vi "Get Server Certificate (Server).vi"(10 "Server Certificates":T1) -> (2 "server certificate file":path)   [LabVIEW 2013, in "OPC UA runtime.lvclass"]
doc: "Get server certificate for OPC UA server connection."
uses:
  OPC UA runtime.lvclass
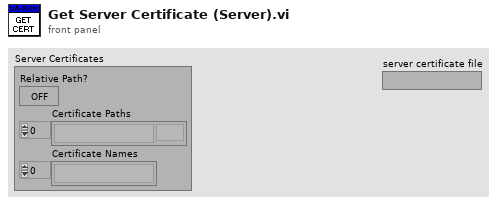
[diagram p1: front panel]
types:
  T1 = cluster{"Relative Path?":bool, "Certificate Paths":path[], "Certificate Names":string[]}
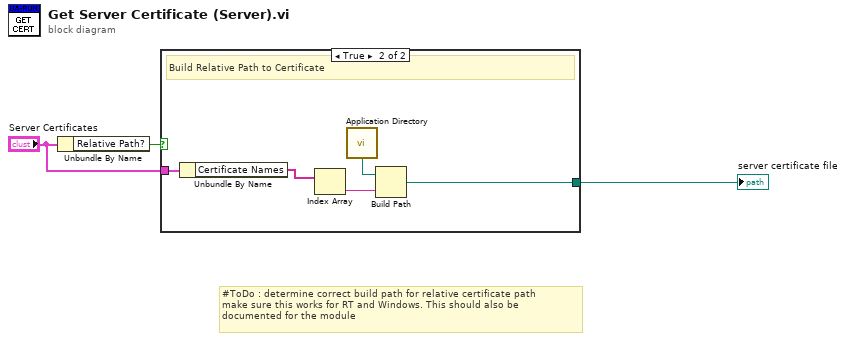
[diagram p0: block diagram]
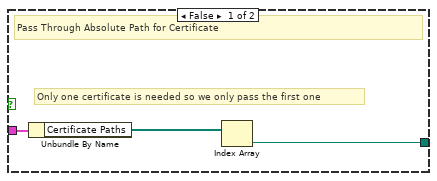
[diagram p2: hidden frame]
diagram:
  # "#ToDo : determine correct build path for relative certificate path\nmake sure this works for RT and Windows. This should also be\ndocumented for the module"
  n1 = Unbundle By Name("Server Certificates") -> ("Relative Path?"=w2:bool)
  n2 = case shown="True" w2 {
    tunnel: "Server Certificates" -> [w6 w11]
    tunnel: [w4 w7] -> w1
    frame False {
      # "Only one certificate is needed so we only pass the first one"
      # "Pass Through Absolute Path for Certificate"
      n3 = Unbundle By Name(w6) -> ("Certificate Paths"=w5:path[])
      n4 = Index Array(array=w5) -> (element=w4:path)  [unwired: 1 in]
    }
    frame True {
      # "Build Relative Path to Certificate"
      n5 = Unbundle By Name(w11) -> ("Certificate Names"=w9:string[])
      n6 = Index Array(array=w9) -> (element=w8:string)  [unwired: 1 in]
      n7 = call <vilib>:"Application Directory.vi"() -> ("Application Directory"=w10:path)
      n8 = Build Path(base path=w10, name or relative path=w8) -> (appended path=w7:path)
    }
  }
  "server certificate file" <- w1
